vi "Initialize.vi"(7 "ChannelName":string="Setpoint.ch%d.SP", 8 "error in":errorcluster, 9 "Number of Channels":u32=1, 10 "Instance Name":string="PluginName", 11 "Setpoint in":refnum<class "Setpoint.lvclass">) -> (0 "error out 2":errorcluster, 2 "Array":string[](array[string]), 3 "Setpoint out":refnum<class "Setpoint.lvclass">)   [LabVIEW 2023, in "Setpoint.lvclass"]
uses:
  Setpoint.lvclass
  Setpoint.lvclass/Setpoint.ctl
  <vilib>/ADAS Replay HIL/Channels/Tag Wrapper/Tag Wrapper.lvlib
  bls-capabilities/src/Capabilities/Utilities/Utilities.lvlib
  <vilib>/ADAS Replay HIL/Channels/Tag Wrapper/Polymorphic/Open Consumer Tag (Double).vi
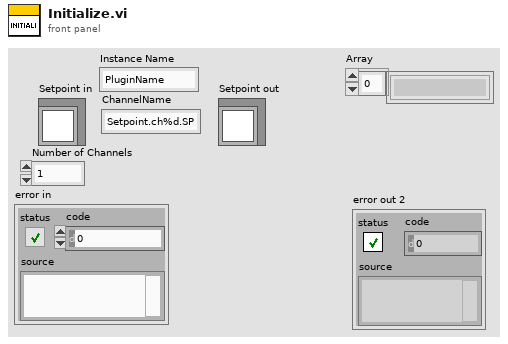
[diagram p1: front panel]
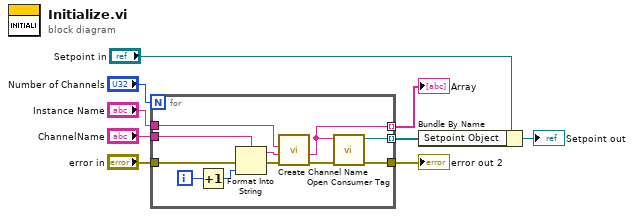
[diagram p0: block diagram]
diagram:
  n1 = for {
    N: "Number of Channels" -> [_]
    tunnel: [w20] -> w9 mode=indexing
    tunnel: [w19] -> w3
    tunnel: "ChannelName" -> [w15]
    tunnel: "Instance Name" -> [w18]
    tunnel: "error in" -> [w11]
    tunnel: [w10] -> w1 mode=indexing
    i -> [w14]
    n2 = Increment(x=w14) -> (x+1=w13:i32)
    n3 = Format Into String(format string=w15, error in=w11, w13) -> (resulting string=w16:string, error out=w12:errorcluster)  [unwired: 1 in]
    n4 = call "Create Channel Name.vi"("error in"=w12, "Channel Name"=w16, "Plugin Name"=w18) -> ("error out"=w17:errorcluster, "Data Channel Name"=w10:string)  [unwired: 7 in]
    n5 = call-poly <vilib>:"Open Consumer Tag.vi"("error in"=w17, "Channel Name"=w10) -> ("error out"=w19:errorcluster, "ADAS HIL Channel"=w20:refnum<k21>)  [unwired: 8 in]
  }
  "error out 2" <- w3
  "Array" <- w1
  n6 = Bundle By Name(cluster="Setpoint in", "Setpoint Object"=w9) -> (→"Setpoint out":refnum<class "Setpoint.lvclass">)
